vi "PH_Strings.Pocketcalculator.vi"(0 "Input":string) -> (1 "String Double":string, 2 "String Integer":string, 3 "Double":dbl, 4 "Integer":i32)   [LabVIEW 2014, in "PH_Common.lvlib"]
doc: "This is a simple calculator. If you just enter a number, this is - rounded in LabVIEW logig! - given out. If you enter something with /, :, x, *, + or -, the VI tries to calculate the result. This only works properly if before and behind the operator a number is given."
uses:
  PH_Common.lvlib
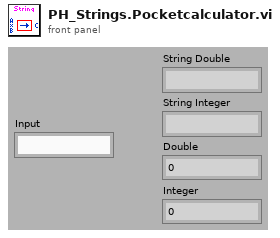
[diagram p1: front panel]
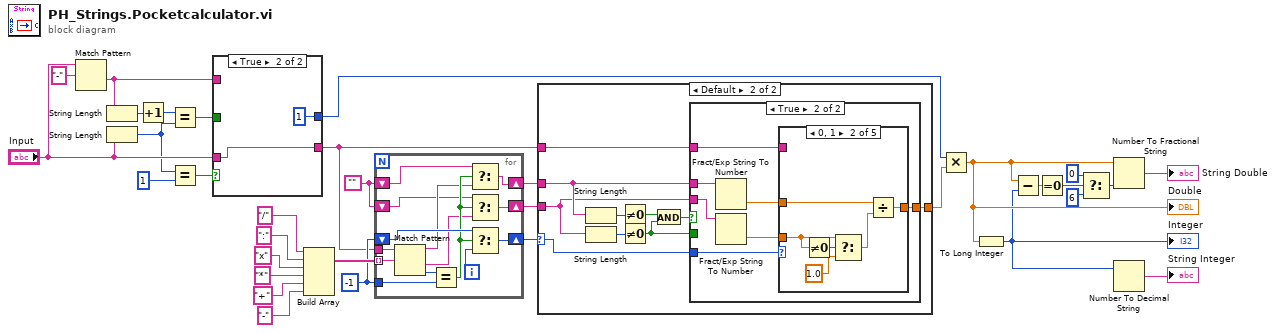
[diagram p0: block diagram]
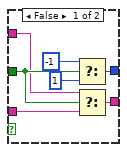
[diagram p2: hidden frame]
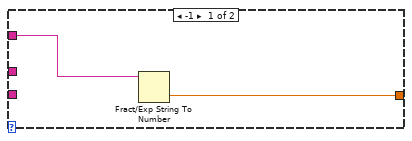
[diagram p3: hidden frame]
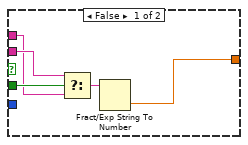
[diagram p4: hidden frame]
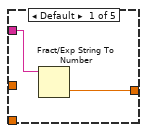
[diagram p5: hidden frame]
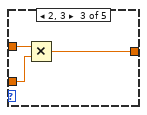
[diagram p6: hidden frame]
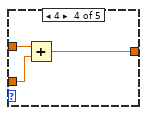
[diagram p7: hidden frame]
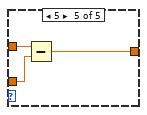
[diagram p8: hidden frame]
diagram:
  w23 = ""
  w20 = -1 ("offset past match")
  n1 = Match Pattern(string="Input", regular expression="-") -> (after substring=w5:string)  [unwired: 1 in, 3 out]
  n2 = String Length(string=w5) -> (length=w18:i32)
  n3 = String Length(string="Input") -> (length=w3:i32)
  n4 = Increment(x=w18) -> (x+1=w17:i32)
  n5 = Equal?(x=w17, y=w3) -> (x = y?=w15:bool)
  n6 = Equal?(x=w3, y=i8 1 ("f")) -> (x = y?=w1:bool)
  n7 = case shown="True" w1 {
    tunnel: [w40 w41] -> w16
    tunnel: w15 -> [w39 _]
    tunnel: [w36 i8 1] -> w14
    tunnel: w5 -> [w35 _]
    tunnel: "Input" -> [w34 w41]
    frame False {
      n8 = Select(t=i8 -1, s=w39, f=i8 1) -> (s? t:f=w36:i8)
      n9 = Select(t=w35, s=w39, f=w34) -> (s? t:f=w40:string)
    }
    frame True {
    }
  }
  n10 = Build Array("/" ("regular expression"), ":" ("element"), "x" ("regular expression"), "*" ("element"), "+" ("regular expression"), "-" ("element")) -> (w29:string[])
  n11 = for {
    tunnel: w16 -> [w56]
    tunnel: w29 -> [w55] mode=indexing
    shift-right: [w52] -> w31
    shift-left: w20 -> [w54]
    shift-right: [w46] -> w22
    shift-left: w23 -> [w49]
    shift-right: [w45] -> w21
    shift-left: w23 -> [w44]
    tunnel: w20 -> [w43]
    i -> [w51]
    n12 = Match Pattern(string=w56, regular expression=w55) -> (before substring=w48:string, after substring=w47:string, offset past match=w53:i32)  [unwired: 1 in, 1 out]
    n13 = Equal?(x=w53, y=w43) -> (x = y?=w50:bool)
    n14 = Select(t=w49, s=w50, f=w48) -> (s? t:f=w46:string)
    n15 = Select(t=w44, s=w50, f=w47) -> (s? t:f=w45:string)
    n16 = Select(t=w54, s=w50, f=w51) -> (s? t:f=w52:i32)
  }
  n17 = case shown="Default" w31 {
    selector: w31 -> [_ w60]
    tunnel: w22 -> [_ w68]
    tunnel: [w58 w67] -> w13
    tunnel: w21 -> [_ w62]
    tunnel: w16 -> [w57 w59]
    frame -1 {
      n18 = Fract/Exp String To Number(string=w57) -> (number=w58:dbl)  [unwired: 3 in, 1 out]
    }
    frame Default {
      n19 = String Length(string=w68) -> (length=w65:i32)
      n20 = String Length(string=w62) -> (length=w66:i32)
      n21 = Not Equal To 0?(x=w65) -> (x != 0?=w64:bool)
      n22 = Not Equal To 0?(x=w66) -> (x != 0?=w61:bool)
      n23 = And(x=w64, y=w61) -> (x .and. y?=w63:bool)
      n24 = case shown="True" w63 {
        tunnel: w68 -> [w69 w80]
        tunnel: w62 -> [w70 w79]
        tunnel: [w73 w77] -> w67
        tunnel: w61 -> [w72 _]
        tunnel: w60 -> [_ w75]
        tunnel: w59 -> [_ w74]
        frame False {
          n25 = Select(t=w70, s=w72, f=w69) -> (s? t:f=w71:string)
          n26 = Fract/Exp String To Number(string=w71) -> (number=w73:dbl)  [unwired: 3 in, 1 out]
        }
        frame True {
          n27 = Fract/Exp String To Number(string=w80) -> (number=w78:dbl)  [unwired: 3 in, 1 out]
          n28 = Fract/Exp String To Number(string=w79) -> (number=w76:dbl)  [unwired: 3 in, 1 out]
          n29 = case shown="0, 1" w75 {
            tunnel: w78 -> [_ w88 w91 w94 w97]
            tunnel: [w81 w87 w90 w93 w96] -> w77
            tunnel: w76 -> [_ w84 w89 w92 w95]
            tunnel: w74 -> [w82 _ _ _ _]
            frame Default {
              n30 = Fract/Exp String To Number(string=w82) -> (number=w81:dbl)  [unwired: 3 in, 1 out]
            }
            frame 0, 1 {
              n31 = Not Equal To 0?(x=w84) -> (x != 0?=w86:bool)
              n32 = Select(t=w84, s=w86, f=1.0) -> (s? t:f=w85:dbl)
              n33 = Divide(x=w88, y=w85) -> (x/y=w87:dbl)
            }
            frame 2, 3 {
              n34 = Multiply(x=w91, y=w89) -> (x*y=w90:dbl)
            }
            frame 4 {
              n35 = Add(x=w94, y=w92) -> (x+y=w93:dbl)
            }
            frame 5 {
              n36 = Subtract(x=w97, y=w95) -> (x-y=w96:dbl)
            }
          }
        }
      }
    }
  }
  n37 = Multiply(x=w14, y=w13) -> (x*y=w12:dbl)
  "Double" <- w12
  n38 = To Long Integer(number=w12) -> (32bit integer=w11:i32)
  "Integer" <- w11
  n39 = Subtract(x=w12, y=w11) -> (x-y=w10:dbl)
  n40 = Equal To 0?(x=w10) -> (x = 0?=w9:bool)
  n41 = Select(t=i16 0 ("precision (6)"), s=w9, f=i16 6) -> (s? t:f=w7:i16)
  n42 = Number To Fractional String(number=w12, precision (6)=w7) -> (F-format string=→"String Double":string)  [unwired: 2 in]
  n43 = Number To Decimal String(number=w11) -> (decimal integer string=→"String Integer":string)  [unwired: 1 in]
